vi "DMA.Add Block (Read).vi"(8 "error in (no error)":errorcluster, 10 "size":u32, 11 "GE 5565PIORC":refnum<class "GE 5565PIORC.lvclass">) -> (0 "error out":errorcluster, 2 "block index":i32, 3 "GE 5565PIORC out":refnum<class "GE 5565PIORC.lvclass">)   [LabVIEW 2016, in "GE 5565PIORC.lvclass"]
uses:
  GE 5565PIORC.lvclass
  Controls/DMA Block Descriptor.ctl
  Controls/DMA Block with Descriptor.ctl
  Controls/DMA Block.ctl
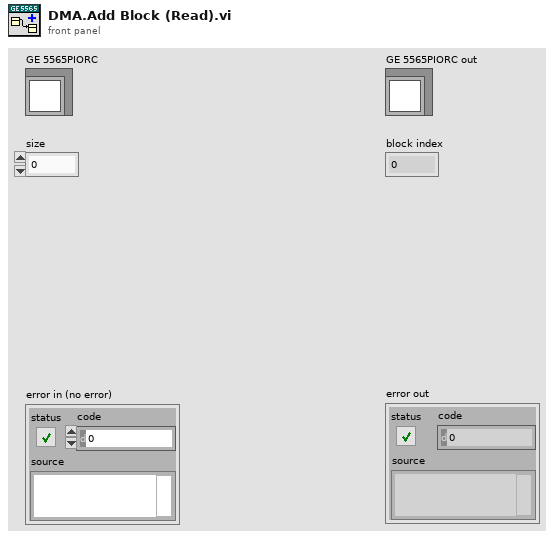
[diagram p1: front panel]
types:
  T1 = typedef "GE 5565PIORC.lvclass/DMA Block with Descriptor.ctl" = cluster{"DMA Block":T2, "Block Descriptor":T3}
  T2 = typedef "GE 5565PIORC.lvclass/DMA Block.ctl" = cluster{"pointer":u32, "size":u32}
  T3 = typedef "GE 5565PIORC.lvclass/DMA Block Descriptor.ctl" = cluster{"descriptor ptr (VISA)":u32, "descriptor size":u32, "descriptor ptr (aligned)":u32, "data ptr (lower)":u32, "data ptr (upper)":u32, "data size":u32, "next descriptor ptr":u32}
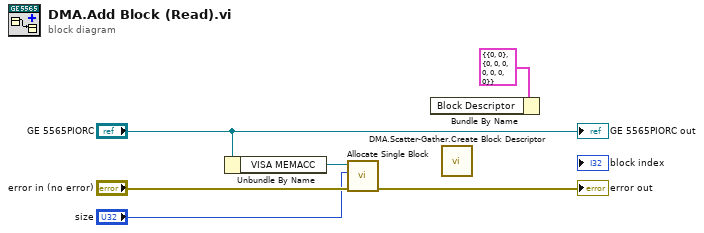
[diagram p0: block diagram]
diagram:
  n1 = Unbundle By Name("GE 5565PIORC") -> ("VISA MEMACC"=w3:refnum<visa-resource-name>)
  n2 = call "Allocate Single Block.vi"("error in (no error)"="error in (no error)", "size (bytes)"="size", "GE 5565PIORC in"=w3) -> ("error out"=→"error out":errorcluster)  [unwired: 6 in, 2 out]
  n3 = Bundle By Name(cluster=T1 {"DMA Block"={"pointer"=0, "size"=0}, "Block Descriptor"={"descriptor ptr (VISA)"=0, "descriptor size"=0, "descriptor ptr (aligned)"=0, "data ptr (lower)"=0, "data ptr (upper)"=0, "data size"=0, "next descriptor ptr"=0}} ("DMA Block with Descriptor")) -> ()  [unwired: 1 in, 1 out]
  n4 = call "DMA.Scatter-Gather.Create Block Descriptor.vi"() -> ()  [unwired: 11 in, 1 out]
  "GE 5565PIORC out" <- "GE 5565PIORC"
